vi "Read View Ref.vi"(8 "error in (no error)":errorcluster, 11 "Debug View In":refnum<class "Debug View.lvclass">) -> (0 "error out":errorcluster, 2 "View Ref":refnum<vi>, 3 "Debug View Out":refnum<class "Debug View.lvclass">)   [LabVIEW 2020, in "Debug View.lvclass"]
uses:
  Debug View.lvclass
  Debug View.lvclass/Debug View.ctl
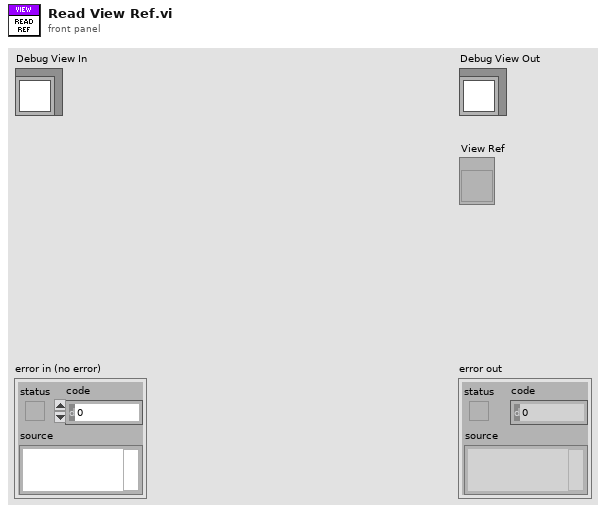
[diagram p1: front panel]
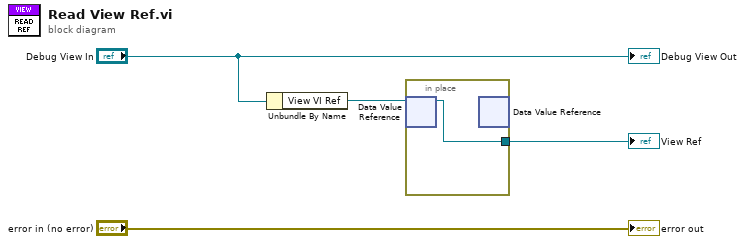
[diagram p0: block diagram]
diagram:
  n1 = Unbundle By Name("Debug View In") -> ("View VI Ref"=w3:refnum<data-value>)
  n2 = in-place {
    in-place-border: [w5] -> w1
    n3 = in-place-dvr #1(w3) -> (w5:refnum<vi>)  [unwired: 1 out]
    n4 = in-place-dvr #1() -> ()  [unwired: 1 in, 2 out]
  }
  "View Ref" <- w1
  "error out" <- "error in (no error)"
  "Debug View Out" <- "Debug View In"
